vi "Create Coverage Report - With Project Files - Reports Package With Same Number of Classes.vi"() -> ()   [LabVIEW 2017, in "Cobertura.Tests.lvlib"]
uses:
  Cobertura.Tests.lvlib
  Fake Code Coverage/Fake Code Coverage.lvclass
  C:/Users/pasca/Projects/Home/lvunit/CodeCoverage/CodeCoverage.lvclass
  Fake Code Inspector/Fake Code Inspector.lvclass
  C:/Users/pasca/Projects/Home/lvunit/Cobertura/Code Inspector Base/Code Inspector Base.lvclass
  Cobertura/Coverage/Coverage.lvclass/Coverage.ctl
  Cobertura/Package/Package.lvclass/Package.ctl
  Cobertura/Coverage/Read Packages.vi
  Cobertura/Package/Read Classes.vi
  Fake Project Inspector/Fake Project Inspector.lvclass
  C:/Users/pasca/Projects/Home/lvunit/Cobertura/Project Inspector Base/Project Inspector Base.lvclass
  Cobertura/Package/Package.lvclass
  Cobertura/Class/Class.lvclass
  Cobertura/Cobertura.lvlib
  <vilib>/PNR/Transparent Assertions/Transparent Assertions/Transparent Assertions.lvlib
  Cobertura/Coverage/Coverage.lvclass
panel:
  out "error out":errorcluster
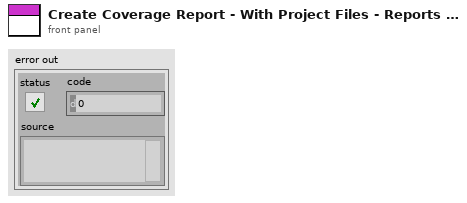
[diagram p1: front panel]
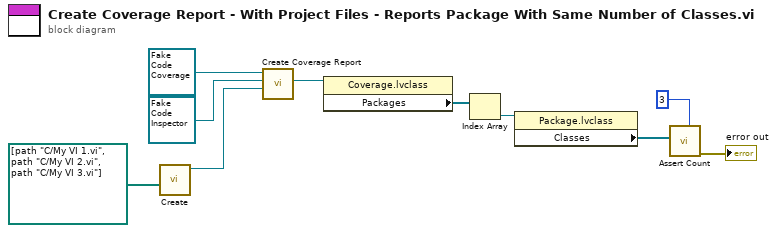
[diagram p0: block diagram]
diagram:
  n1 = call "Create.vi"("Item Paths"=path[] [path "C:/My VI 1.vi", path "C:/My VI 2.vi", path "C:/My VI 3.vi"]) -> ("Fake Project Inspector"=w5:refnum<class "Fake Project Inspector.lvclass">)  [unwired: 9 in, 1 out]
  n2 = call "Create Coverage Report.vi"("Project Inspector"=w5, "Code Inspector"=refnum<class "Fake Code Inspector.lvclass"> refnum ("Cobertura.Tests.lvlib:Fake Code Inspector.lvclass"), "CodeCoverage in"=refnum<class "Fake Code Coverage.lvclass"> refnum ("Cobertura.Tests.lvlib:Fake Code Coverage.lvclass")) -> ("Coverage"=w10:refnum<class "Coverage.lvclass">)  [unwired: 7 in, 1 out]
  n3 = property class="Coverage.lvclass"(reference=w10) -> ("Packages"=w8:refnum<class "Package.lvclass">[])  [unwired: 1 in, 2 out]
  n4 = Index Array(array=w8) -> (element=w2:refnum<class "Package.lvclass">)  [unwired: 1 in]
  n5 = property class="Package.lvclass"(reference=w2) -> ("Classes"=w1:refnum<class "Class.lvclass">[])  [unwired: 1 in, 2 out]
  n6 = call <vilib>:"Assert Count.vi"("Expected"=3, "Haystack"=w1) -> ("error out"=→"error out":errorcluster)  [unwired: 9 in]
